vi "Lab Panel V5.40.vi"() -> ()   [LabVIEW 2017]
uses:
  sub vi/SelectLAB0X-N.ctl
  sub vi/SIG LAB0X-N.ctl
  sub vi/Set LAB0X-N.ctl
  <vilib>/Platform/TimedLoop/XDataNode/timing_clust.ctl
  <vilib>/Platform/TimedLoop/XDataNode/nitl_modes.ctl
  <vilib>/Platform/TimedLoop/XDataNode/wakeup.ctl
  Global display 1.vi
  Global display 4.vi
  Global display 3.vi
  Global display 2.vi
  Global 1.vi
  <vilib>/platform/TimedLoop/XDataNode/XDataNode.xnode
  <vilib>/Platform/TimedLoop/XDataNode/XDNodeRunTimeDep.lvlib
panel:
  in  "path to JPEG file":path=path "C:/Users/Mike/Documents/Crabtree/Crabtree/Hardware/crabtree"
  out "Simulate IND":bool
  out "Amb Tp":dbl format="%#.0f"
  out "Tp Up":dbl
  out "network error":bool
  out "TEMP":bool
  out "AI":bool
  in  "stop all":bool
  in  "ADMIN":bool
  in  "Tab Control 2":T1(tab)
  out "SIG LAB05-2":T2 {"PF" format="%.2f"; "AMPS" format="%.1f"}
  out "SIG LAB05-1":T2 {"PF" format="%.2f"; "AMPS" format="%.1f"}
  out "SIG LAB04-2":T2 {"PF" format="%.2f"; "AMPS" format="%.1f"}
  out "SIG LAB04-1":T2 {"PF" format="%.2f"; "AMPS" format="%.1f"}
  out "SIG LAB03-2":T2 {"PF" format="%.2f"; "AMPS" format="%.1f"}
  out "SIG LAB03-1":T2 {"PF" format="%.2f"; "AMPS" format="%.1f"}
  out "SIG LAB02-2":T2 {"PF" format="%.2f"; "AMPS" format="%.1f"}
  in  "RUN LAB01-1":bool
  in  "O/I  LAB05-1":bool
  in  "O/I  LAB05-2":bool
  in  "O/I  LAB04-1":bool
  in  "O/I  LAB04-2":bool
  in  "O/I  LAB02-1":bool
  in  "O/I  LAB02-2":bool
  in  "O/I  LAB01-2":bool
  in  "O/I  LAB01-1":bool
  in  "O/I  LAB03-1":bool
  in  "RUN LAB05-2":bool
  in  "RUN LAB05-1":bool
  in  "RUN LAB04-2":bool
  in  "RUN LAB04-1":bool
  in  "RUN LAB03-2":bool
  in  "RUN LAB03-1":bool
  in  "RUN LAB02-2":bool
  in  "RUN LAB02-1":bool
  in  "RUN LAB01-2":bool
  in  "SELECT LAB05-2":T3
  in  "SELECT LAB05-1":T3
  in  "SELECT LAB04-2":T3
  in  "SELECT LAB04-1":T3
  in  "SELECT LAB03-2":T3
  in  "SELECT LAB03-1":T3
  in  "SELECT LAB02-2":T3
  in  "SELECT LAB02-1":T3
  in  "SELECT LAB01-2":T3
  in  "SELECT LAB01-1":T3
  in  "O/I  LAB03-2":bool
  out "SIG LAB01-1":T2 {"PF" format="%.2f"; "AMPS" format="%.1f"}
  out "SIG LAB01-2":T2 {"PF" format="%.2f"; "AMPS" format="%.1f"}
  out "SIG LAB02-1":T2 {"PF" format="%.2f"; "AMPS" format="%.1f"}
  out "DISP LAB05-2":T4 {"MINS" format="%.2g"}
  out "DISP LAB05-1":T4 {"MINS" format="%.2g"}
  out "DISP LAB04-2":T4 {"MINS" format="%.2g"}
  out "DISP LAB04-1":T4 {"MINS" format="%.2g"}
  out "DISP LAB03-2":T4 {"MINS" format="%.2g"}
  out "DISP LAB03-1":T4 {"MINS" format="%.2g"}
  in  "SET LAB05-2":T5={"NAME"="", "DESCRIPTION"="", "CYCLES"=5.0, "T-RISE mins"=0.0, "T-RISE deg C"=0.0} {"CYCLES" min=5.0 step=1.0}
  in  "SET LAB05-1":T5={"NAME"="", "DESCRIPTION"="", "CYCLES"=5.0, "T-RISE mins"=0.0, "T-RISE deg C"=0.0} {"CYCLES" min=5.0 step=1.0}
  in  "SET LAB04-2":T5={"NAME"="", "DESCRIPTION"="", "CYCLES"=5.0, "T-RISE mins"=0.0, "T-RISE deg C"=0.0} {"CYCLES" min=5.0 step=1.0}
  in  "SET LAB04-1":T5={"NAME"="", "DESCRIPTION"="", "CYCLES"=5.0, "T-RISE mins"=0.0, "T-RISE deg C"=0.0} {"CYCLES" min=5.0 step=1.0}
  in  "SET LAB03-2":T5={"NAME"="", "DESCRIPTION"="", "CYCLES"=5.0, "T-RISE mins"=0.0, "T-RISE deg C"=0.0} {"CYCLES" min=5.0 step=1.0}
  in  "SET LAB03-1":T5={"NAME"="", "DESCRIPTION"="", "CYCLES"=5.0, "T-RISE mins"=0.0, "T-RISE deg C"=0.0} {"CYCLES" min=5.0 step=1.0}
  out "DISP LAB02-2":T4 {"MINS" format="%.2g"}
  out "DISP LAB02-1":T4 {"MINS" format="%.2g"}
  in  "SET LAB02-2":T5={"NAME"="", "DESCRIPTION"="", "CYCLES"=5.0, "T-RISE mins"=0.0, "T-RISE deg C"=0.0} {"CYCLES" min=5.0 step=1.0}
  in  "SET LAB02-1":T5={"NAME"="", "DESCRIPTION"="", "CYCLES"=5.0, "T-RISE mins"=0.0, "T-RISE deg C"=0.0} {"CYCLES" min=5.0 step=1.0}
  out "RESULT LAB05-2":bool
  out "RESULT LAB05-1":bool
  out "RESULT LAB04-2":bool
  out "RESULT LAB04-1":bool
  out "RESULT LAB03-2":bool
  out "RESULT LAB03-1":bool
  out "RESULT LAB02-2":bool
  out "RESULT LAB02-1":bool
  out "RESULT LAB01-2":bool
  out "RESULT LAB01-1":bool
  in  "SET LAB01-1":T6={"NAME"="", "DESCRIPTION"="", "CYCLES"=5.0, "T-RISE mins"=0.0, "T-RISE deg C"=0.0} {"CYCLES" min=5.0 step=1.0}
  in  "SET LAB01-2":T5={"NAME"="", "DESCRIPTION"="", "CYCLES"=5.0, "T-RISE mins"=0.0, "T-RISE deg C"=0.0} {"CYCLES" min=5.0 step=1.0}
  out "DISP LAB01-1":T4 {"MINS" format="%.2g"}
  out "DISP LAB01-2":T4 {"MINS" format="%.2f"}
  out "TEMP RISE LAB05-2":cluster{"TL":dbl, "TN":dbl}
  out "TEMP RISE LAB05-1":cluster{"TL":dbl, "TN":dbl}
  out "TEMP RISE LAB04-2":cluster{"TL":dbl, "TN":dbl}
  out "TEMP RISE LAB04-1":cluster{"TL":dbl, "TN":dbl}
  out "TEMP RISE LAB03-2":cluster{"TL":dbl, "TN":dbl}
  out "TEMP RISE LAB03-1":cluster{"TL":dbl, "TN":dbl}
  out "TEMP RISE LAB02-2":cluster{"TL":dbl, "TN":dbl}
  out "TEMP RISE LAB02-1":cluster{"TL":dbl, "TN":dbl}
  out "TEMP RISE LAB01-2":cluster{"TL":dbl, "TN":dbl}
  out "TEMP RISE LAB01-1":cluster{"TL":dbl, "TN":dbl}
  out "JIG LAB05-2":bool
  out "JIG LAB05-1":bool
  out "JIG LAB04-2":bool
  out "JIG LAB04-1":bool
  out "JIG LAB03-2":bool
  out "JIG LAB03-1":bool
  out "JIG LAB02-2":bool
  out "JIG LAB02-1":bool
  out "JIG LAB01-2":bool
  out "JIG LAB01-1":bool
  out "TEMP START LAB01-1":cluster{"TL":dbl, "TN":dbl}
  out "TEMP START LAB02-1":cluster{"TL":dbl, "TN":dbl}
  out "TEMP START LAB03-1":cluster{"TL":dbl, "TN":dbl}
  out "TEMP START LAB04-1":cluster{"TL":dbl, "TN":dbl}
  out "TEMP START LAB01-2":cluster{"TL":dbl, "TN":dbl}
  out "TEMP START LAB02-2":cluster{"TL":dbl, "TN":dbl}
  out "TEMP START LAB03-2":cluster{"TL":dbl, "TN":dbl}
  out "TEMP START LAB04-2":cluster{"TL":dbl, "TN":dbl}
  out "TEMP START LAB05-2":cluster{"TL":dbl, "TN":dbl}
  out "TEMP START LAB05-1":cluster{"TL":dbl, "TN":dbl}
  out "LOG LAB05-2":string
  out "LOG LAB04-2":string
  out "LOG LAB03-2":string
  out "LOG LAB02-2":string
  out "LOG LAB01-2":string
  out "LOG LAB05-1":string
  out "LOG LAB04-1":string
  out "LOG LAB03-1":string
  out "LOG LAB02-1":string
  out "LOG LAB01-1":string
  in  "Tab charts":T7(tab)
  out "LAB01 VOLTS":dynamicdata(graph)
  out "LAB01 AMPS":dynamicdata(graph)
  out "LAB01 deg C":dynamicdata(graph)
  out "LAB02 VOLTS":dynamicdata(graph)
  out "LAB02 AMPS":dynamicdata(graph)
  out "LAB02 deg C":dynamicdata(graph)
  out "LAB03 VOLTS":dynamicdata(graph)
  out "LAB03 AMPS":dynamicdata(graph)
  out "LAB03 deg C":dynamicdata(graph)
  out "LAB04 VOLTS":dynamicdata(graph)
  out "LAB04 AMPS":dynamicdata(graph)
  out "LAB04 deg C":dynamicdata(graph)
  out "LAB05 VOLTS":dynamicdata(graph)
  out "LAB05 AMPS":dynamicdata(graph)
  out "LAB05 deg C":dynamicdata(graph)
  out "Reset Error":bool
  out "Er USB#2":dbl
  out "Er USB#1":dbl
  out "Er USB#0":dbl
  out "Resets Done":dbl
  out "Error USB #2":bool
  out "Error USB #1":bool
  out "Error USB #0":bool
  in  "MAIL SETTINGS":T8
  out "MAIL REPORT":string
  in  "TO (string):":string
  in  "Send Mail Now":bool
  in  "Auto Mail Send":bool
  in  "Network Directory":path
  in  "JIG ON TIME (S)":dbl=1.0 min=1.0 max=10.0 step=0.5 format="%.1g"
  in  "JIG OFF TIME (S)":dbl=2.0 min=2.0 max=10.0 step=0.5 format="%.1g"
  in  "Reset Measuring":bool
  out "JIG RELAY CYCLES":T9
  out "ON L05-2":cluster{"amps":dbl, "volts":dbl, "pf":dbl}
  out "ON L05-1":cluster{"amps":dbl, "volts":dbl, "pf":dbl}
  out "FAIL LAB05-2":cluster{"LO":dbl, "HI":dbl}
  out "FAIL LAB05-1":cluster{"LO":dbl, "HI":dbl}
  out "FAIL LAB04-2":cluster{"LO":dbl, "HI":dbl}
  out "FAIL LAB04-1":cluster{"LO":dbl, "HI":dbl}
  out "FAIL LAB03-2":cluster{"LO":dbl, "HI":dbl}
  out "FAIL LAB03-1":cluster{"LO":dbl, "HI":dbl}
  out "FAIL LAB02-2":cluster{"LO":dbl, "HI":dbl}
  out "FAIL LAB02-1":cluster{"LO":dbl, "HI":dbl}
  out "FAIL LAB01-2":cluster{"LO":dbl, "HI":dbl}
  out "FAIL LAB01-1":cluster{"LO":dbl, "HI":dbl}
  out "ON L01-1":cluster{"amps":dbl, "volts":dbl, "pf":dbl}
  out "ON L01-2":cluster{"amps":dbl, "volts":dbl, "pf":dbl}
  out "ON L02-1":cluster{"amps":dbl, "volts":dbl, "pf":dbl}
  out "ON L02-2":cluster{"amps":dbl, "volts":dbl, "pf":dbl}
  out "ON L03-1":cluster{"amps":dbl, "volts":dbl, "pf":dbl}
  out "ON L03-2":cluster{"amps":dbl, "volts":dbl, "pf":dbl}
  out "ON L04-1":cluster{"amps":dbl, "volts":dbl, "pf":dbl}
  out "ON L04-2":cluster{"amps":dbl, "volts":dbl, "pf":dbl}
  in  "Open Com Port":bool
  out "LA05-2 (TN)":bool
  out "LA05-2 (TL)":bool
  out "LA05-1 (TN)":bool
  out "LA05-1 (TL)":bool
  out "LA04-2 (TN)":bool
  out "LA04-2 (TL)":bool
  out "LA04-1 (TN)":bool
  out "LA04-1 (TL)":bool
  out "LA03-2 (TN)":bool
  out "LA03-2 (TL)":bool
  out "LA03-1 (TN)":bool
  out "LA03-1 (TL)":bool
  out "LA02-2 (TN)":bool
  out "LA02-2 (TL)":bool
  out "LA02-1 (TN)":bool
  out "LA02-1 (TL)":bool
  out "LA01-2 (TN)":bool
  out "LA01-2 (TL)":bool
  out "LA01-1 (TN)":bool
  out "LA01-1 (TL)":bool
  out "TEMP LA05":T10
  out "TEMP LA04":T10
  out "TEMP LA03":T10
  out "TEMP LA02":T10
  out "TEMP LA01":T10
  out "Ref deg C":dbl format="%#.0f"
  out "Temp read loop":dbl
  out "Com Port Status":bool
  out "Com setup loops":i32
  out "VISA Com out":refnum<visa-resource-name>
  in  "Select COM port":refnum<visa-resource-name>="COM6"
  in  "Read Temp":bool
  out "Error Temp":bool
  out "AI Task":bool
  out "AI Task2":dbl
  out "AI Task1":dbl
  out "AI Task0":dbl
  out "Total USB resets":dbl
  in  "Auto Reset":bool
  in  "Mail Test File To:":string
  in  "Mail Test Fail":bool
  out "graph flag":bool
  in  "Temp Test Cal":dbl
  in  "Amps Fail level":dbl
  in  "Fail Loops":dbl
  out "Save JC":bool
  in  "Simulate":bool
  in  "Temp Value":dbl
  in  "Temp Delay Lps":dbl
  in  "SAMPLES":dbl
  in  "RATE (Hz)":dbl
  in  "JIG TEST":T11
  in  "C drive data root dir":path
  out "run lab05-2":bool
  out "run lab05-1":bool
  out "run lab04-2":bool
  out "run lab04-1":bool
  out "run lab03-2":bool
  out "run lab03-1":bool
  out "run lab02-2":bool
  out "run lab02-1":bool
  out "run lab01-2":bool
  out "run lab01-1":bool
  in  "Tab Control":T12(tab)
  out "LAB01-2 (GRAPH)":dynamicdata(graph)
  out "LAB01-1 (GRAPH)":dynamicdata(graph)
  out "LAB02-2 (GRAPH)":dynamicdata(graph)
  out "LAB02-1 (GRAPH)":dynamicdata(graph)
  out "LAB03-2 (GRAPH)":dynamicdata(graph)
  out "LAB03-1 (GRAPH)":dynamicdata(graph)
  out "LAB04-2 (GRAPH)":dynamicdata(graph)
  out "LAB04-1 (GRAPH)":dynamicdata(graph)
  out "LAB05-2 (GRAPH)":dynamicdata(graph)
  out "LAB05-1 (GRAPH)":dynamicdata(graph)
  out "Any Test Running":bool
  out "Read Time":dbl
  out "LAB05 TEMP":T13
  out "LAB04 TEMP":T13
  out "LAB02 TEMP":T13
  out "LAB01 TEMP":T13
  out "LAB03 TEMP":T13
  out "LAB05-TP":bool
  out "LAB04-TP":bool
  out "LAB03-TP":bool
  out "LAB02-TP":bool
  out "LAB01-TP":bool
  out "Analog error":bool
  out "USB OUT 0":bool[](array[boolean])
  out "USB OUT 1":bool[](array[boolean])
  out "USB OUT 2":bool[](array[boolean])
  in  "Ambient Volts":dbl format="%.2f"
  in  "PF":dbl min=0.0 max=1.0 step=0.1 format="%#.1f"
  in  "VOLTS":dbl
  in  "OFF amps":dbl min=0.0 max=100.0 step=0.1 format="%#.1f"
  in  "ON amps":dbl
  in  "LAB deg C":T14
  out "AI data 0":waveform(dbl)[](array[waveform])
  out "AI data 1":waveform(dbl)[](array[waveform])
  out "AI data 2":waveform(dbl)[](array[waveform])
  out "AI Error":errorcluster[](array[cluster])
  out "AI loop time":dbl format="%.6g"
  out "loops":dbl
  out "on loops":dbl format="%#.0f"
  out "off loops":dbl format="%#.0f"
  out "jig cycle":dbl
  out "TDMS LAB01-1":refnum<k34>
  out "data file error":errorcluster
  out "TDMS LAB02-1":refnum<k34>
  out "TDMS LAB01-2":refnum<k34>
  out "TDMS LAB02-2":refnum<k34>
  out "TDMS LAB03-1":refnum<k34>
  out "TDMS LAB03-2":refnum<k34>
  out "TDMS LAB04-1":refnum<k34>
  out "TDMS LAB04-2":refnum<k34>
  out "TDMS LAB05-1":refnum<k34>
  out "TDMS LAB05-2":refnum<k34>
  out "mail control":string
  out "File Time Stamp":timestamp
  in  "stop":bool
  out "deg C (volts)":dbl
  out "TEMP REF cal":dbl
  out "CAL LAB01":T15 {"2 (TN) cal" min=0.0 step=0.01 format="%.2f"; "2 (TL) cal" min=0.0 step=0.01 format="%.2f"; "2 (PF) cal" min=0.0 step=0.01 format="%.2f"; "2 (V) cal" min=0.0 step=0.01 format="%.2f"; "2 (A) cal" min=0.0 step=0.01 format="%.2f"; "1 (TN) cal" min=0.0 step=0.01 format="%.2f"; "1 (TL) cal" min=0.0 step=0.01 format="%.2f"; "1 (PF) cal" min=0.0 step=0.01 format="%.2f"; "1 (V) cal" min=0.0 step=0.01 format="%.2f"; "1  (A) cal" min=0.0 step=0.01 format="%.2f"}
  out "CAL LAB03":T15 {"2 (TN) cal" min=0.0 step=0.01 format="%.2f"; "2 (TL) cal" min=0.0 step=0.01 format="%.2f"; "2 (PF) cal" min=0.0 step=0.01 format="%.2f"; "2 (V) cal" min=0.0 step=0.01 format="%.2f"; "2 (A) cal" min=0.0 step=0.01 format="%.2f"; "1 (TN) cal" min=0.0 step=0.01 format="%.2f"; "1 (TL) cal" min=0.0 step=0.01 format="%.2f"; "1 (PF) cal" min=0.0 step=0.01 format="%.2f"; "1 (V) cal" min=0.0 step=0.01 format="%.2f"; "1  (A) cal" min=0.0 step=0.01 format="%.2f"}
  out "CAL LAB02":T16 {"2 (TN) cal" min=0.0 step=0.01 format="%.2f"; "2 (TL) cal" min=0.0 step=0.01 format="%.2f"; "2 (PF) cal" min=0.0 step=0.01 format="%.2f"; "2 (V) cal" min=0.0 step=0.01 format="%.2f"; "2 (A) cal" min=0.0 step=0.01 format="%.2f"; "1 (TN) cal" min=0.0 step=0.01 format="%.2f"; "1 (TL) cal" min=0.0 step=0.01 format="%.2f"; "1 (PF) cal" min=0.0 step=0.01 format="%.2f"; "1 (V) cal" min=0.0 step=0.01 format="%.2f"; "1 (A) cal" min=0.0 step=0.01 format="%.2f"}
  out "CAL LAB05":T15 {"2 (TN) cal" min=0.0 step=0.01 format="%.2f"; "2 (TL) cal" min=0.0 step=0.01 format="%.2f"; "2 (PF) cal" min=0.0 step=0.01 format="%.2f"; "2 (V) cal" min=0.0 step=0.01 format="%.2f"; "2 (A) cal" min=0.0 step=0.01 format="%.2f"; "1 (TN) cal" min=0.0 step=0.01 format="%.2f"; "1 (TL) cal" min=0.0 step=0.01 format="%.2f"; "1 (PF) cal" min=0.0 step=0.01 format="%.2f"; "1 (V) cal" min=0.0 step=0.01 format="%.2f"; "1  (A) cal" min=0.0 step=0.01 format="%.2f"}
  out "CAL LAB04":T15 {"2 (TN) cal" min=0.0 step=0.01 format="%.2f"; "2 (TL) cal" min=0.0 step=0.01 format="%.2f"; "2 (PF) cal" min=0.0 step=0.01 format="%.2f"; "2 (V) cal" min=0.0 step=0.01 format="%.2f"; "2 (A) cal" min=0.0 step=0.01 format="%.2f"; "1 (TN) cal" min=0.0 step=0.01 format="%.2f"; "1 (TL) cal" min=0.0 step=0.01 format="%.2f"; "1 (PF) cal" min=0.0 step=0.01 format="%.2f"; "1 (V) cal" min=0.0 step=0.01 format="%.2f"; "1  (A) cal" min=0.0 step=0.01 format="%.2f"}
  out "cal file error out":errorcluster
  in  "SET (cal)":bool
  out "AI Data 0":waveform(dbl)[](graph)
  out "AI Data 1":waveform(dbl)[](graph)
  out "AI Data 2":waveform(dbl)[](graph)
  # "LAB01"
  # "LAB02"
  # "LAB03"
  # "LAB04"
  # "LAB05"
  # "LAB01"
  # "LAB02"
  # "LAB03"
  # "LAB04"
  # "LAB05"
  # "PANEL ID / DATE / TIME / NAME / DESCRIPTION / CYCLES / TEST TIME / STATUS"
  # "PANEL ID / DATE / TIME / NAME / DESCRIPTION / CYCLES / TEST TIME / STATUS"
  # "(Enter recipients address seperated by comma)"
  # "JIG SET"
  # "Temperature circuits \ndetected at start up."
  # "PANEL CONTROL TO BE ON"
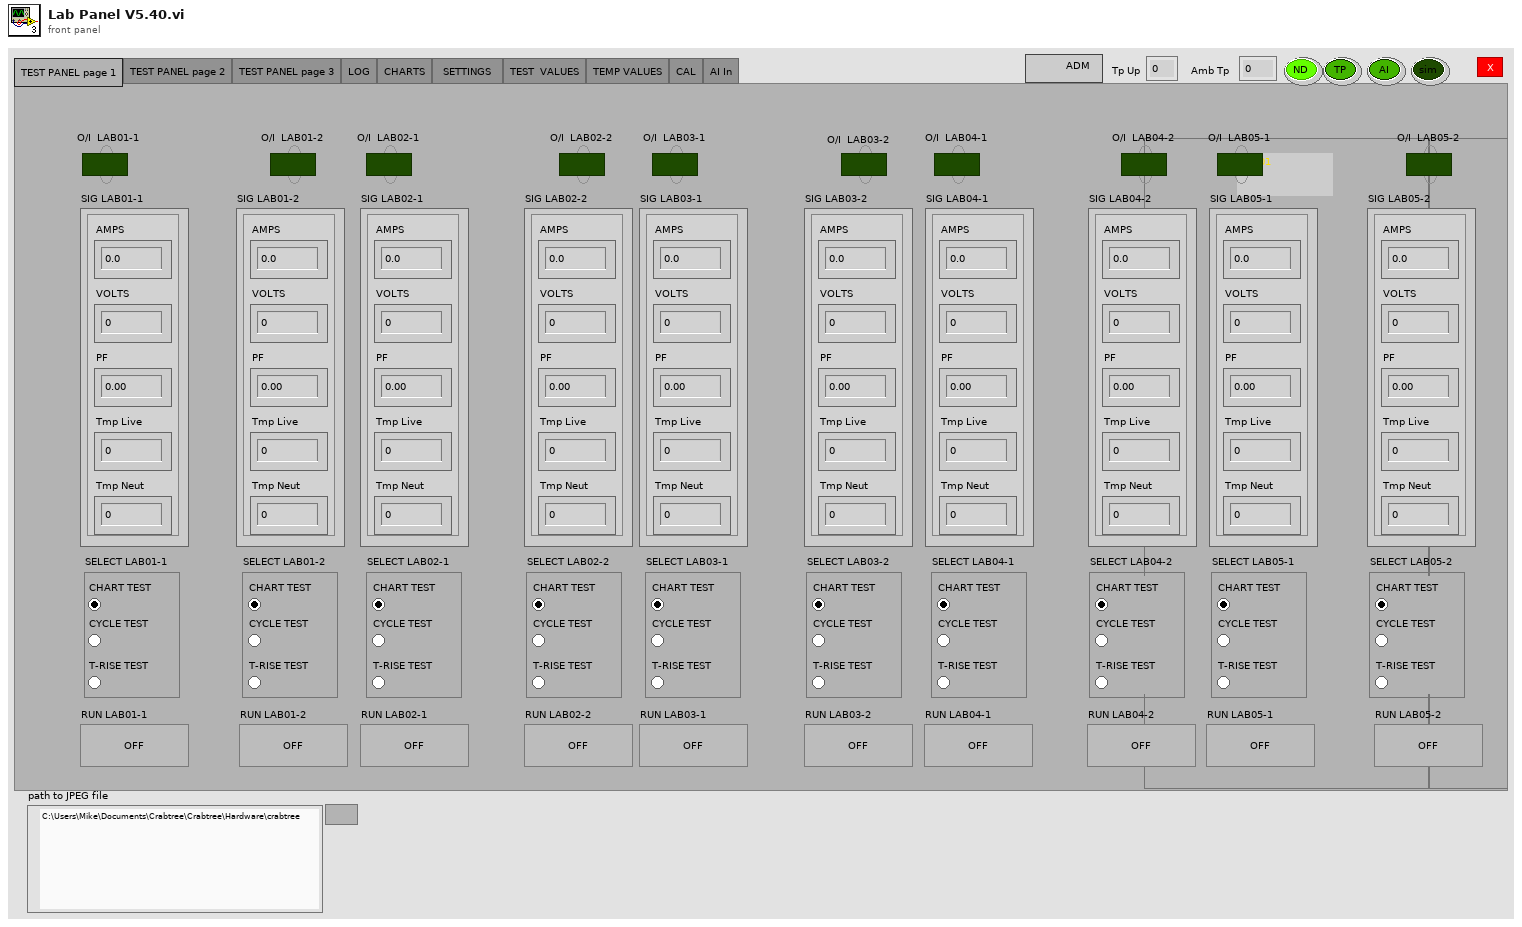
[diagram p1: front panel]
types:
  T1 = enum32{"TEST PANEL page 1", "TEST PANEL page 2", "TEST PANEL page 3", "LOG", "CHARTS", "SETTINGS   ", "TEST  VALUES", "TEMP VALUES", "ADM", "CAL", "AI In"}
  T2 = typedef "SIG LAB0X-N.ctl" = cluster{"AMPS":dbl, "VOLTS":dbl, "PF":dbl, "Tmp Live":dbl, "Tmp Neut":dbl}
  T3 = typedef "SelectLAB0X-N.ctl" = enum32{"CHART TEST", "CYCLE TEST", "T-RISE TEST"}
  T4 = cluster{"CYCLE":dbl, "MINS":dbl, "STATUS":string}
  T5 = cluster{"NAME":string, "DESCRIPTION":string, "CYCLES":dbl, "T-RISE mins":dbl, "T-RISE deg C":dbl}
  T6 = typedef "Set LAB0X-N.ctl" = cluster{"NAME":string, "DESCRIPTION":string, "CYCLES":dbl, "T-RISE mins":dbl, "T-RISE deg C":dbl}
  T7 = enum32{"LAB01", "LAB02", "LAB03", "LAB04", "LAB05"}
  T8 = cluster{"OUT SERVER ADDRESS":string, "FROM ACCOUNT":string, "USER NAME":string, "PASSWORD":string, "TEST MAIL":bool, "TEST MAIL STATUS":string, "mail error":errorcluster}
  T9 = cluster{"LAB01-1":dbl, "LAB01-2":dbl, "LAB02-1":dbl, "LAB02-2":dbl, "LAB03-1":dbl, "LAB03-2":dbl, "LAB04-1":dbl, "LAB04-2":dbl, "LAB05-1":dbl, "LAB05-2":dbl}
  T10 = cluster{"TL-1":dbl, "TN-1":dbl, "TL-2":dbl, "TN-2":dbl, "TL -1COUNT":dbl, "TN-1 COUNT":dbl, "TL-2 COUNT":dbl, "TN-2 COUNT":dbl}
  T11 = cluster{" LAB01-1":bool, " LAB01-2":bool, "LAB02-1":bool, " LAB02-2":bool, "LAB03-1":bool, "LAB03-2":bool, "LAB04-1":bool, "LAB04-2":bool, "LAB05-1":bool, "LAB05-2":bool}
  T12 = enum32{"LAB01", "LAB02", "LAB03", "LAB04", "LAB05", "TEMPERATURE", "GENERAL INFO", "Simulate", "AI Data Out"}
  T13 = cluster{"T1 Live":dbl, "T1 Neut":dbl, "T2 Live":dbl, "T2 Neut":dbl, "ID":dbl, "ER":dbl}
  T14 = cluster{"1 TL":dbl, "1 TN":dbl, "2 TL":dbl, "2 TN":dbl, "ID":dbl, "ER":dbl}
  T15 = cluster{"1  (A) cal":dbl, "1 (V) cal":dbl, "1 (PF) cal":dbl, "1 (TL) cal":dbl, "1 (TN) cal":dbl, "2 (A) cal":dbl, "2 (V) cal":dbl, "2 (PF) cal":dbl, "2 (TL) cal":dbl, "2 (TN) cal":dbl}
  T16 = cluster{"1 (A) cal":dbl, "1 (V) cal":dbl, "1 (PF) cal":dbl, "1 (TL) cal":dbl, "1 (TN) cal":dbl, "2 (A) cal":dbl, "2 (V) cal":dbl, "2 (PF) cal":dbl, "2 (TL) cal":dbl, "2 (TN) cal":dbl}
  T17 = enum8{"Enabled", "Disabled", "Disabled and Grayed Out"}
  T18 = enum16{"open", "replace", "create", "open or create", "replace or create", "replace or create with confirmation"}
  T19 = typedef "XDNodeRunTimeDep.lvlib/timing_clust.ctl" = cluster{"Expected End [f-1]":u64, "Actual End [f-1]":u64, "Finished Late? [f-1]":bool, "Expected End [i-1]":u64, "Actual End [i-1]":u64, "Finished Late? [i-1]":bool, "Expected Start [i]":u64, "Actual Start [i]":u64, "Expected Start [f]":u64, "Actual Start [f]":u64, "Source Name":string, "Structure Name":string, "Period":i64, "Deadline":i64, "Offset":i64, "Start":i64, "Priority":i32, "Timeout":i32, "Mode":T20, "Wakeup Reason":T21, "Error":errorcluster, "Source Type":string, "Secondary Source Type":string, "Global End Time":u64, "Global Start Time":u64, "Frame Duration":u64, "Iteration Duration":u64, "Assigned CPU":i32, "I/O Scan Engine Mode":u32}
  T20 = typedef "XDNodeRunTimeDep.lvlib/nitl_modes.ctl" = enum32{"No Change", "Process missed periods, maintain original phase", "Discard missed periods, maintain original phase", "Process missed periods, ignore original phase", "Discard missed periods, ignore original phase"}
  T21 = typedef "XDNodeRunTimeDep.lvlib/wakeup.ctl" = enum32{"Normal", "Aborted", "Asynchronous wakeup", "Timing source error", "Timed loop error", "Timeout"}
  T22 = enum16{"open", "open or create", "create or replace", "create", "open (read-only)"}
  T23 = cluster{"status":string, "mail server":string, "mail from":string, "mail to":string, "mail file":bool}
  T24 = cluster{"SET LAB01-1":T6, "SET LAB01-2":cluster{"NAME":string, "DESCRIPTION":string, "CYCLES":dbl, "T-RISE mins":dbl, "T-RISE deg C":dbl}, "SET LAB02-1":cluster{"NAME":string, "DESCRIPTION":string, "CYCLES":dbl, "T-RISE mins":dbl, "T-RISE deg C":dbl}, "SET LAB02-2":cluster{"NAME":string, "DESCRIPTION":string, "CYCLES":dbl, "T-RISE mins":dbl, "T-RISE deg C":dbl}, "SET LAB03-1":cluster{"NAME":string, "DESCRIPTION":string, "CYCLES":dbl, "T-RISE mins":dbl, "T-RISE deg C":dbl}, "SET LAB03-2":cluster{"NAME":string, "DESCRIPTION":string, "CYCLES":dbl, "T-RISE mins":dbl, "T-RISE deg C":dbl}, "SET LAB04-1":cluster{"NAME":string, "DESCRIPTION":string, "CYCLES":dbl, "T-RISE mins":dbl, "T-RISE deg C":dbl}, "SET LAB04-2":cluster{"NAME":string, "DESCRIPTION":string, "CYCLES":dbl, "T-RISE mins":dbl, "T-RISE deg C":dbl}, "SET LAB05-1":cluster{"NAME":string, "DESCRIPTION":string, "CYCLES":dbl, "T-RISE mins":dbl, "T-RISE deg C":dbl}, "SET LAB05-2":cluster{"NAME":string, "DESCRIPTION":string, "CYCLES":dbl, "T-RISE mins":dbl, "T-RISE deg C":dbl}, "Network Directory":path, "C drive data root dir":path, "RATE (Hz)":dbl, "SAMPLES":dbl, "Select COM port":refnum<visa-resource-name>, "Temp Delay Lps":dbl, "Temp Value":dbl, "Fail Loops":dbl, "Temp Test Cal":dbl, "Amps Fail level":dbl, "Mail Test File To:":string, "Mail Test Fail":bool}
  T25 = cluster{"MAIL SETTINGS":cluster{"OUT SERVER ADDRESS":string, "FROM ACCOUNT":string, "USER NAME":string, "PASSWORD":string, "TEST MAIL":bool, "TEST MAIL STATUS":string, "mail error":errorcluster}, "Auto Mail Send":bool, string}
  T26 = cluster{"id1":bool, "id2":bool, "id3":bool, "id4":bool, "id5":bool}
  T27 = cluster{"T1":dbl, "T2":dbl, "T3":dbl, "T4":dbl, "ID":dbl, "ER":dbl}
  T28 = typedef "imagedata.ctl" = cluster{"image type":i32, "image depth":i32, "image":u8[], "mask":u8[], "colors":u32[], "Rectangle":cluster{"left":i16, "top":i16, "right":i16, "bottom":i16}}
  T29 = cluster{"STATUS":string, "OUT SERVER ADDRESS":string, "FROM ACCOUNT":string, "Mail Test File To:":string, "Mail Test Fail":bool}
  T30 = cluster{"LAB01-1 (A)":dbl, "LAB01-1 (V)":dbl, "LAB01-1 (PF)":dbl, "LAB01-2 (A)":dbl, "LAB01-2 (V)":dbl, "LAB01-2 (PF)":dbl}
  T31 = cluster{"LAB02-1 (A)":dbl, "LAB02-1 (V)":dbl, "LAB02-1 (PF)":dbl, "LAB02-2 (A)":dbl, "LAB02-2 (V)":dbl, "LAB02-2 (PF)":dbl}
  T32 = cluster{"LAB03-1 (A)":dbl, "LAB03-1 (V)":dbl, "LAB03-1 (PF)":dbl, "LAB03-2 (A)":dbl, "LAB03-2 (V)":dbl, "LAB03-2 (PF)":dbl}
  T33 = cluster{"LAB04-1 (A)":dbl, "LAB04-1 (V)":dbl, "LAB04-1 (PF)":dbl, "LAB04-2 (A)":dbl, "LAB04-2 (V)":dbl, "LAB04-2 (PF)":dbl}
  T34 = cluster{"LAB05-1 (A)":dbl, "LAB05-1 (V)":dbl, "LAB05-1 (PF)":dbl, "LAB05-2 (A)":dbl, "LAB05-2 (V)":dbl, "LAB05-2 (PF)":dbl}
  T35 = cluster{"OFF amps":dbl, "VOLTS":dbl, "PF":dbl, "OFF amps":dbl, "VOLTS":dbl, "PF":dbl}
  T36 = cluster{"FAIL LAB01-1":cluster{"LO":dbl, "HI":dbl}, "SIG LAB01-1":T2, "TEMP START LAB01-1":cluster{"TL":dbl, "TN":dbl}, "DISP LAB01-1":cluster{"CYCLE":dbl, "MINS":dbl, "STATUS":string}, "SET LAB01-1":T6, "TDMS LAB01-1":refnum<k34>}
  T37 = cluster{"FAIL LAB01-2":cluster{"LO":dbl, "HI":dbl}, "SIG LAB01-2":T2, "TEMP START LAB01-2":cluster{"TL":dbl, "TN":dbl}, "DISP LAB01-2":cluster{"CYCLE":dbl, "MINS":dbl, "STATUS":string}, "SET LAB01-2":cluster{"NAME":string, "DESCRIPTION":string, "CYCLES":dbl, "T-RISE mins":dbl, "T-RISE deg C":dbl}, "TDMS LAB01-2":refnum<k34>}
  T38 = cluster{"FAIL LAB02-1":cluster{"LO":dbl, "HI":dbl}, "SIG LAB02-1":T2, "TEMP START LAB02-1":cluster{"TL":dbl, "TN":dbl}, "DISP LAB02-1":cluster{"CYCLE":dbl, "MINS":dbl, "STATUS":string}, "SET LAB02-1":cluster{"NAME":string, "DESCRIPTION":string, "CYCLES":dbl, "T-RISE mins":dbl, "T-RISE deg C":dbl}, "TDMS LAB02-1":refnum<k34>}
  T39 = cluster{"FAIL LAB02-2":cluster{"LO":dbl, "HI":dbl}, "SIG LAB02-2":T2, "TEMP START LAB02-2":cluster{"TL":dbl, "TN":dbl}, "DISP LAB02-2":cluster{"CYCLE":dbl, "MINS":dbl, "STATUS":string}, "SET LAB02-2":cluster{"NAME":string, "DESCRIPTION":string, "CYCLES":dbl, "T-RISE mins":dbl, "T-RISE deg C":dbl}, "TDMS LAB02-2":refnum<k34>}
  T40 = cluster{"FAIL LAB03-1":cluster{"LO":dbl, "HI":dbl}, "SIG LAB03-1":T2, "TEMP START LAB03-1":cluster{"TL":dbl, "TN":dbl}, "DISP LAB03-1":cluster{"CYCLE":dbl, "MINS":dbl, "STATUS":string}, "SET LAB03-1":cluster{"NAME":string, "DESCRIPTION":string, "CYCLES":dbl, "T-RISE mins":dbl, "T-RISE deg C":dbl}, "TDMS LAB03-1":refnum<k34>}
  T41 = cluster{"FAIL LAB03-2":cluster{"LO":dbl, "HI":dbl}, "SIG LAB03-2":T2, "TEMP START LAB03-2":cluster{"TL":dbl, "TN":dbl}, "DISP LAB03-2":cluster{"CYCLE":dbl, "MINS":dbl, "STATUS":string}, "SET LAB03-2":cluster{"NAME":string, "DESCRIPTION":string, "CYCLES":dbl, "T-RISE mins":dbl, "T-RISE deg C":dbl}, "TDMS LAB03-2":refnum<k34>}
  T42 = cluster{"FAIL LAB04-1":cluster{"LO":dbl, "HI":dbl}, "SIG LAB04-1":T2, "TEMP START LAB04-1":cluster{"TL":dbl, "TN":dbl}, "DISP LAB04-1":cluster{"CYCLE":dbl, "MINS":dbl, "STATUS":string}, "SET LAB04-1":cluster{"NAME":string, "DESCRIPTION":string, "CYCLES":dbl, "T-RISE mins":dbl, "T-RISE deg C":dbl}, "TDMS LAB04-1":refnum<k34>}
  T43 = cluster{"FAIL LAB04-2":cluster{"LO":dbl, "HI":dbl}, "SIG LAB04-2":T2, "TEMP START LAB04-2":cluster{"TL":dbl, "TN":dbl}, "DISP LAB04-2":cluster{"CYCLE":dbl, "MINS":dbl, "STATUS":string}, "SET LAB04-2":cluster{"NAME":string, "DESCRIPTION":string, "CYCLES":dbl, "T-RISE mins":dbl, "T-RISE deg C":dbl}, "TDMS LAB04-2":refnum<k34>}
  T44 = cluster{"FAIL LAB05-1":cluster{"LO":dbl, "HI":dbl}, "SIG LAB05-1":T2, "TEMP START LAB05-1":cluster{"TL":dbl, "TN":dbl}, "DISP LAB05-1":cluster{"CYCLE":dbl, "MINS":dbl, "STATUS":string}, "SET LAB05-1":cluster{"NAME":string, "DESCRIPTION":string, "CYCLES":dbl, "T-RISE mins":dbl, "T-RISE deg C":dbl}, "TDMS LAB05-1":refnum<k34>}
  T45 = cluster{"FAIL LAB05-2":cluster{"LO":dbl, "HI":dbl}, "SIG LAB05-2":T2, "TEMP START LAB05-2":cluster{"TL":dbl, "TN":dbl}, "DISP LAB05-2":cluster{"CYCLE":dbl, "MINS":dbl, "STATUS":string}, "SET LAB05-2":cluster{"NAME":string, "DESCRIPTION":string, "CYCLES":dbl, "T-RISE mins":dbl, "T-RISE deg C":dbl}, "TDMS LAB05-2":refnum<k34>}
  T46 = cluster{"MAIL SETTINGS":cluster{"OUT SERVER ADDRESS":string, "FROM ACCOUNT":string, "USER NAME":string, "PASSWORD":string, "TEST MAIL":bool, "TEST MAIL STATUS":string, "mail error":errorcluster}, "Auto Mail Send":bool, "TO (string):":string}
  T47 = cluster{"TP1-L":dbl, "TP1-N":dbl, "TP2-L":dbl, "TP2-N":dbl, "TP1-L COUNT":dbl, "TP1-N COUNT":dbl, "TP2-L COUNT":dbl, "TP2-N COUNT":dbl}
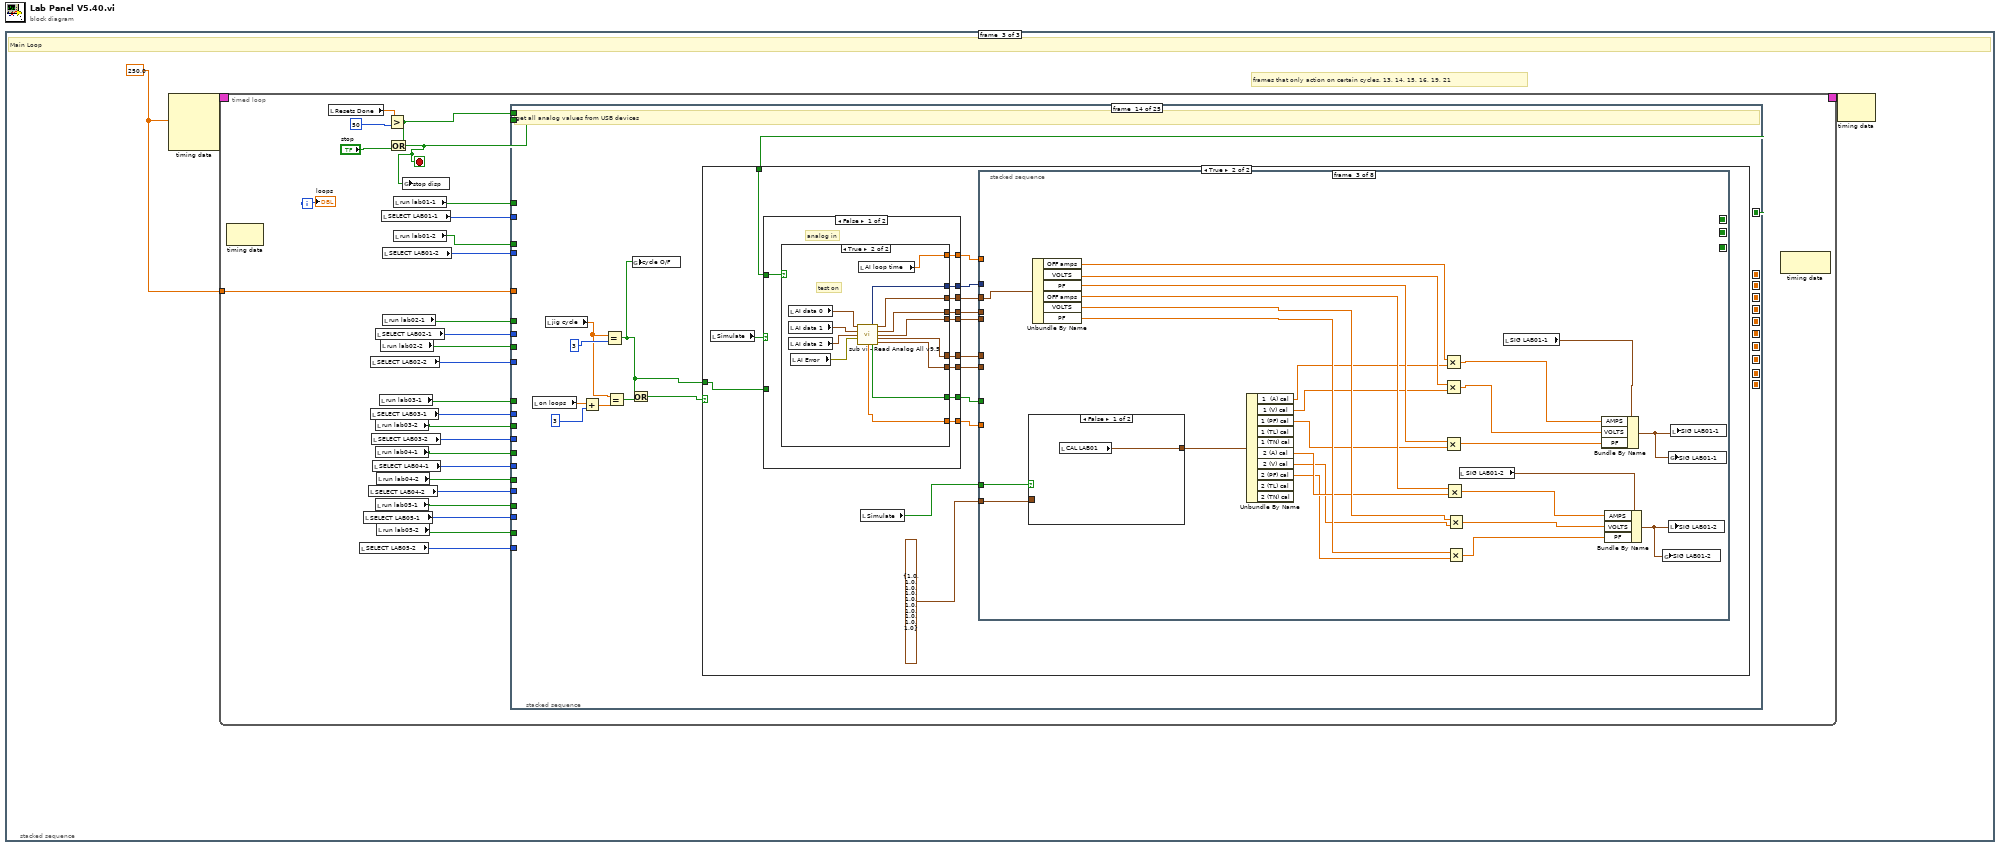
[diagram p0: block diagram]
diagram:
  n1 = stacked-sequence {
    frame #0 {
      n2 = local write "Save JC"(FALSE) -> ()
      "jig cycle" <- 0
    }
    frame #1 {
      # "do 1st time set up"
      n3 = stacked-sequence {
        frame #0 {
          # "check for simulate mode"
          n4 = call "subvi-simulate v1.vi"() -> ("Sim"=w3:bool)  [unwired: 11 in]
          n5 = case shown="True" w3 {
            frame False {
            }
            frame True {
              n6 = local write "Simulate"(TRUE) -> ()
            }
          }
        }
        frame #1 {
          # "RESET USB AND TEMPERATURE CIRCUITS"
          n7 = local read "Simulate"() -> (w5:bool)
          n8 = case shown="False" w5 {
            frame False {
              n9 = call "Reset USB&temp v 1.vi"() -> ()  [unwired: 11 in, 1 out]
            }
            frame True {
            }
          }
        }
        frame #2 {
          # "Disable front panel while 1st time set up is being done"
          n10 = disable-structure shown="Enabled" {
            frame Enabled {
              n11 = property on="Tab Control 2" class="TabCtl (strict)"() -> ("Pages"=w12:refnum<vi>[])  [unwired: 2 in, 2 out]
              n12 = Index Array(array=w12, index=8) -> (element=w10:refnum<vi>)
              n13 = property class="Page"(reference=w10, "PageVis"=FALSE) -> ()  [unwired: 1 in, 2 out]
            }
            frame Disabled {
            }
          }
          n14 = property on="Tab Control 2" class="TabCtl (strict)"("Value"=0) -> ()  [unwired: 2 in, 2 out]
          n15 = local write "ADMIN"(FALSE) -> ()
          n16 = property on="Tab Control 2" class="TabCtl (strict)"("DisabledEnum"=T17."Disabled and Grayed Out" ("Disabled")) -> ()  [unwired: 2 in, 2 out]
        }
        frame #3 {
          # "Get calibration values"
          n17 = call "sub vi - get calibration values v1.vi"() -> ("TEMP REF CAL"=w13:dbl, "LAB01 (CAL)"=→"CAL LAB01":T15, "LAB02 (CAL)"=→"CAL LAB02":T16, "LAB03 (CAL)"=→"CAL LAB03":T15, "LAB04 (CAL)"=→"CAL LAB04":T15, "calibration file error out"=→"cal file error out":errorcluster, "LAB05 (CAL)"=→"CAL LAB05":T15)  [unwired: 9 in]
          n18 = local write "TEMP REF cal"(w13) -> ()
        }
        frame #4 {
          # "get last saved test settings from file"
          n19 = local read "Network Directory"() -> (w42:path)
          n20 = local read "C drive data root dir"() -> (w40:path)
          n21 = local read "SET LAB05-2"() -> (w72:T5)
          n22 = local read "SAMPLES"() -> (w38:dbl)
          n23 = local read "SET LAB05-1"() -> (w73:T5)
          n24 = local read "RATE (Hz)"() -> (w39:dbl)
          n25 = local read "SET LAB04-2"() -> (w74:T5)
          n26 = local read "SET LAB03-2"() -> (w71:T5)
          n27 = local read "SET LAB04-1"() -> (w75:T5)
          n28 = local read "SET LAB03-1"() -> (w70:T5)
          n29 = local read "SET LAB02-2"() -> (w69:T5)
          n30 = local read "SET LAB02-1"() -> (w68:T5)
          n31 = local read "SET LAB01-2"() -> (w67:T5)
          n32 = local read "SET LAB01-1"() -> (w66:T6)
          n33 = local read "Select COM port"() -> (w35:refnum<visa-resource-name>)
          n34 = local read "Temp Delay Lps"() -> (w34:dbl)
          n35 = local read "Mail Test File To:"() -> (w24:string)
          n36 = local read "Temp Value"() -> (w33:dbl)
          n37 = local read "Temp Test Cal"() -> (w28:dbl)
          n38 = local read "Amps Fail level"() -> (w27:dbl)
          n39 = local read "Fail Loops"() -> (w30:dbl)
          n40 = local read "Mail Test Fail"() -> (w22:bool)
          n41 = Bundle("SET LAB01-1"=w66, "SET LAB01-2"=w67, "SET LAB02-1"=w68, "SET LAB02-2"=w69, "SET LAB03-1"=w70, "SET LAB03-2"=w71, "SET LAB04-1"=w75, "SET LAB04-2"=w74, "SET LAB05-1"=w73, "SET LAB05-2"=w72, "Network Directory"=w42, "C drive data root dir"=w40, "RATE (Hz)"=w39, "SAMPLES"=w38, "Select COM port"=w35, "Temp Delay Lps"=w34, "Temp Value"=w33, "Fail Loops"=w30, "Temp Test Cal"=w28, "Amps Fail level"=w27, "Mail Test File To:"=w24, "Mail Test Fail"=w22) -> (w59:T24)  [unwired: 1 in]
          n42 = String To Path(string="c:\\crabtree\\Set Up\\") -> (path=w63:path)
          n43 = Build Path(base path=w63, name or relative path="settings.bin") -> (appended path=w61:path)
          n44 = Create Folder(path (use dialog)=w63) -> (error out=w65:errorcluster)  [unwired: 2 in, 2 out]
          n45 = call <vilib>:"Clear Errors.vi"("error in (no error)"=w65) -> ()  [unwired: 5 in, 2 out]
          n46 = Open/Create/Replace File(file path (use dialog)=w61) -> (refnum out=w58:refnum<file>, error out=w60:errorcluster)  [unwired: 5 in, 1 out]
          n47 = Read from Binary File(5:w59, 8:w60, 11:w58) -> (0:w55:errorcluster, 2:w57:T24, 3:w56:refnum<file>)  [unwired: 3 in, 1 out]
          n48 = Unbundle(w57) -> ("SET LAB01-1"=w53:T6, "SET LAB01-2"=w52:T5, "SET LAB02-1"=w51:T5, "SET LAB02-2"=w50:T5, "SET LAB03-1"=w49:T5, "SET LAB03-2"=w48:T5, "SET LAB04-1"=w47:T5, "SET LAB04-2"=w46:T5, "SET LAB05-1"=w45:T5, "SET LAB05-2"=w44:T5, "Network Directory"=w43:path, "C drive data root dir"=w41:path, "RATE (Hz)"=w36:dbl, "SAMPLES"=w37:dbl, "Select COM port"=w20:refnum<visa-resource-name>, "Temp Delay Lps"=w32:dbl, "Temp Value"=w31:dbl, "Fail Loops"=w29:dbl, "Temp Test Cal"=w26:dbl, "Amps Fail level"=w25:dbl, "Mail Test File To:"=w23:string, "Mail Test Fail"=w21:bool)
          n49 = Close File(refnum=w56, error in=w55) -> (error out=w54:errorcluster)  [unwired: 1 out]
          n50 = local write "data file error"(w54) -> ()
          n51 = local write "Temp Test Cal"(w26) -> ()
          n52 = local write "Amps Fail level"(w25) -> ()
          n53 = local write "Mail Test File To:"(w23) -> ()
          n54 = local write "Mail Test Fail"(w21) -> ()
          n55 = local write "Fail Loops"(w29) -> ()
          n56 = local write "Temp Delay Lps"(w32) -> ()
          n57 = local write "C drive data root dir"(w41) -> ()
          n58 = local write "Temp Value"(w31) -> ()
          n59 = local write "Network Directory"(w43) -> ()
          n60 = local write "SAMPLES"(w37) -> ()
          n61 = local write "RATE (Hz)"(w36) -> ()
          n62 = local write "SET LAB04-2"(w46) -> ()
          n63 = local write "SET LAB05-1"(w45) -> ()
          n64 = local write "SET LAB04-1"(w47) -> ()
          n65 = local write "SET LAB05-2"(w44) -> ()
          n66 = local write "SET LAB02-1"(w51) -> ()
          n67 = local write "SET LAB02-2"(w50) -> ()
          n68 = local write "SET LAB03-1"(w49) -> ()
          n69 = local write "SET LAB03-2"(w48) -> ()
          n70 = local write "SET LAB01-1"(w53) -> ()
          n71 = local write "SET LAB01-2"(w52) -> ()
          n72 = local write "Select COM port"(w20) -> ()
          n73 = global write "Global 1.vi" "COM port"(w20) -> ()
        }
        frame #5 {
          # "Get total resets value from file"
          n74 = String To Path(string="c:\\crabtree\\Set Up\\") -> (path=w86:path)
          n75 = Build Path(base path=w86, name or relative path="USB resets.bin") -> (appended path=w79:path)
          n76 = Create Folder(path (use dialog)=w86) -> (error out=w78:errorcluster)  [unwired: 2 in, 2 out]
          n77 = call <vilib>:"Clear Errors.vi"("error in (no error)"=w78) -> ()  [unwired: 5 in, 2 out]
          n78 = Open/Create/Replace File(file path (use dialog)=w79, operation (0:open)=T18."open or create") -> (refnum out=w84:refnum<file>, error out=w83:errorcluster)  [unwired: 4 in, 1 out]
          n79 = local read "Total USB resets"() -> (w77:dbl)
          n80 = Read from Binary File(5:w77, 8:w83, 11:w84) -> (0:w81:errorcluster, 2:w76:dbl, 3:w82:refnum<file>)  [unwired: 3 in, 1 out]
          n81 = local write "Total USB resets"(w76) -> ()
          n82 = Close File(refnum=w82, error in=w81) -> (error out=w80:errorcluster)  [unwired: 1 out]
          n83 = local write "data file error"(w80) -> ()
        }
        frame #6 {
          # "Get last saved jig cycles value from file"
          n84 = String To Path(string="c:\\crabtree\\Jig Cycles\\") -> (path=w98:path)
          n85 = Build Path(base path=w98, name or relative path="jigcycles.bin") -> (appended path=w96:path)
          n86 = Create Folder(path (use dialog)=w98) -> (error out=w100:errorcluster)  [unwired: 2 in, 2 out]
          n87 = call <vilib>:"Clear Errors.vi"("error in (no error)"=w100) -> ()  [unwired: 5 in, 2 out]
          n88 = Open/Create/Replace File(file path (use dialog)=w96) -> (refnum out=w94:refnum<file>, error out=w95:errorcluster)  [unwired: 5 in, 1 out]
          n89 = Read from Binary File(5:T9 {"LAB01-1"=0.0, "LAB01-2"=0.0, "LAB02-1"=0.0, "LAB02-2"=0.0, "LAB03-1"=0.0, "LAB03-2"=0.0, "LAB04-1"=0.0, "LAB04-2"=0.0, "LAB05-1"=0.0, "LAB05-2"=0.0} ("JIG RELAY CYCLES"), 8:w95, 11:w94) -> (0:w92:errorcluster, 2:w89:T9, 3:w93:refnum<file>)  [unwired: 3 in, 1 out]
          n90 = local write "JIG RELAY CYCLES"(w89) -> ()
          n91 = Close File(refnum=w93, error in=w92) -> (error out=w91:errorcluster)  [unwired: 1 out]
          n92 = local write "data file error"(w91) -> ()
        }
        frame #7 {
          # "Get mail settings"
          n93 = local read "Auto Mail Send"() -> (w104:bool)
          n94 = local read "MAIL SETTINGS"() -> (w108:T8)
          n95 = String To Path(string="c:\\crabtree\\Set Up\\") -> (path=w116:path)
          n96 = Build Path(base path=w116, name or relative path="mail.bin") -> (appended path=w114:path)
          n97 = Create Folder(path (use dialog)=w116) -> (error out=w118:errorcluster)  [unwired: 2 in, 2 out]
          n98 = Bundle("MAIL SETTINGS"=w108, "Auto Mail Send"=w104, "") -> (w107:T25)  [unwired: 1 in]
          n99 = call <vilib>:"Clear Errors.vi"("error in (no error)"=w118) -> ()  [unwired: 5 in, 2 out]
          n100 = Open/Create/Replace File(file path (use dialog)=w114) -> (refnum out=w112:refnum<file>, error out=w113:errorcluster)  [unwired: 5 in, 1 out]
          n101 = Read from Binary File(5:w107, 8:w113, 11:w112) -> (0:w110:errorcluster, 2:w106:T25, 3:w111:refnum<file>)  [unwired: 3 in, 1 out]
          n102 = Unbundle(w106) -> ("MAIL SETTINGS"=w105:T8, "Auto Mail Send"=w103:bool, w102:string)
          n103 = local write "Auto Mail Send"(w103) -> ()
          n104 = local write "TO (string):"(w102) -> ()
          n105 = local write "MAIL SETTINGS"(w105) -> ()
          n106 = Close File(refnum=w111, error in=w110) -> (error out=w109:errorcluster)  [unwired: 1 out]
          n107 = local write "data file error"(w109) -> ()
        }
        frame #8 {
          # "Set display status if blank"
          n108 = local read "DISP LAB03-2"() -> (w148:T4)
          n109 = local read "DISP LAB03-1"() -> (w155:T4)
          n110 = local read "DISP LAB02-2"() -> (w162:T4)
          n111 = local read "DISP LAB01-2"() -> (w175:T4)
          n112 = local read "DISP LAB01-1"() -> (w184:T4)
          n113 = local read "DISP LAB02-1"() -> (w169:T4)
          n114 = Unbundle(w148) -> ("STATUS"=w150:string)  [unwired: 2 out]
          n115 = Unbundle(w155) -> ("STATUS"=w157:string)  [unwired: 2 out]
          n116 = Unbundle(w162) -> ("STATUS"=w164:string)  [unwired: 2 out]
          n117 = Unbundle(w169) -> ("STATUS"=w171:string)  [unwired: 2 out]
          n118 = Unbundle(w175) -> ("STATUS"=w178:string)  [unwired: 2 out]
          n119 = Unbundle(w184) -> ("STATUS"=w185:string)  [unwired: 2 out]
          n120 = Equal?(x="", y=w150) -> (x = y?=w152:bool)
          n121 = Equal?(x="", y=w157) -> (x = y?=w159:bool)
          n122 = Equal?(x="", y=w164) -> (x = y?=w166:bool)
          n123 = Equal?(x="", y=w171) -> (x = y?=w173:bool)
          n124 = Equal?(x="", y=w178) -> (x = y?=w180:bool)
          n125 = Equal?(x="", y=w185) -> (x = y?=w187:bool)
          n126 = Select(t="STOP", s=w152, f=w150) -> (s? t:f=w149:string)
          n127 = Select(t="STOP", s=w159, f=w157) -> (s? t:f=w156:string)
          n128 = Select(t="STOP", s=w166, f=w164) -> (s? t:f=w163:string)
          n129 = Select(t="STOP", s=w173, f=w171) -> (s? t:f=w170:string)
          n130 = Select(t="STOP", s=w180, f=w178) -> (s? t:f=w177:string)
          n131 = Select(t="STOP", s=w187, f=w185) -> (s? t:f=w183:string)
          n132 = Bundle(cluster=w148, "STATUS"=w149) -> (w147:T4)  [unwired: 2 in]
          n133 = Bundle(cluster=w155, "STATUS"=w156) -> (w154:T4)  [unwired: 2 in]
          n134 = Bundle(cluster=w162, "STATUS"=w163) -> (w161:T4)  [unwired: 2 in]
          n135 = Bundle(cluster=w169, "STATUS"=w170) -> (w168:T4)  [unwired: 2 in]
          n136 = Bundle(cluster=w175, "STATUS"=w177) -> (w176:T4)  [unwired: 2 in]
          n137 = Bundle(cluster=w184, "STATUS"=w183) -> (w182:T4)  [unwired: 2 in]
          n138 = local write "DISP LAB01-2"(w176) -> ()
          n139 = local write "DISP LAB01-1"(w182) -> ()
          n140 = local write "DISP LAB02-1"(w168) -> ()
          n141 = local write "DISP LAB03-1"(w154) -> ()
          n142 = local write "DISP LAB02-2"(w161) -> ()
          n143 = local write "DISP LAB03-2"(w147) -> ()
          n144 = local read "DISP LAB05-2"() -> (w120:T4)
          n145 = local read "DISP LAB05-1"() -> (w127:T4)
          n146 = local read "DISP LAB04-2"() -> (w129:T4)
          n147 = local read "DISP LAB04-1"() -> (w131:T4)
          n148 = Unbundle(w120) -> ("STATUS"=w122:string)  [unwired: 2 out]
          n149 = Unbundle(w127) -> ("STATUS"=w133:string)  [unwired: 2 out]
          n150 = Unbundle(w129) -> ("STATUS"=w138:string)  [unwired: 2 out]
          n151 = Unbundle(w131) -> ("STATUS"=w143:string)  [unwired: 2 out]
          n152 = Equal?(x="", y=w122) -> (x = y?=w124:bool)
          n153 = Equal?(x="", y=w133) -> (x = y?=w135:bool)
          n154 = Equal?(x="", y=w138) -> (x = y?=w140:bool)
          n155 = Equal?(x="", y=w143) -> (x = y?=w145:bool)
          n156 = Select(t="STOP", s=w124, f=w122) -> (s? t:f=w121:string)
          n157 = Select(t="STOP", s=w135, f=w133) -> (s? t:f=w132:string)
          n158 = Select(t="STOP", s=w140, f=w138) -> (s? t:f=w137:string)
          n159 = Select(t="STOP", s=w145, f=w143) -> (s? t:f=w142:string)
          n160 = Bundle(cluster=w120, "STATUS"=w121) -> (w119:T4)  [unwired: 2 in]
          n161 = Bundle(cluster=w127, "STATUS"=w132) -> (w126:T4)  [unwired: 2 in]
          n162 = Bundle(cluster=w129, "STATUS"=w137) -> (w128:T4)  [unwired: 2 in]
          n163 = Bundle(cluster=w131, "STATUS"=w142) -> (w130:T4)  [unwired: 2 in]
          n164 = local write "DISP LAB05-2"(w119) -> ()
          n165 = local write "DISP LAB05-1"(w126) -> ()
          n166 = local write "DISP LAB04-1"(w130) -> ()
          n167 = local write "DISP LAB04-2"(w128) -> ()
        }
        frame #9 {
          w192 = 0
          w189 = FALSE
          # "initialise analog error control"
          n168 = local write "Resets Done"(0) -> ()
          n169 = local write "Auto Reset"(TRUE) -> ()
          n170 = local write "Er USB#0"(w192) -> ()
          n171 = local write "Er USB#1"(w192) -> ()
          n172 = local write "Er USB#2"(w192) -> ()
          n173 = local write "Analog error"(w189) -> ()
          n174 = local write "Reset Measuring"(w189) -> ()
          n175 = local write "Error USB #0"(w189) -> ()
          n176 = local write "Reset Error"(w189) -> ()
          n177 = local write "Error USB #1"(w189) -> ()
          n178 = local write "Error USB #2"(w189) -> ()
          n179 = local write "stop"(w189) -> ()
          n180 = local write "stop all"(w189) -> ()
        }
        frame #10 {
          # "get initial temperature values"
          n181 = stacked-sequence {
            frame #0 {
              w201 = T13 {"T1 Live"=20.0, "T1 Neut"=20.0, "T2 Live"=20.0, "T2 Neut"=20.0, "ID"=6.0, "ER"=10.0} ("LAB01 TEMP")
              n182 = local read "Select COM port"() -> (w196:refnum<visa-resource-name>)
              n183 = local write "LAB deg C"(w201) -> ()
              n184 = global write "Global display 4.vi" "LAB deg C"(w201) -> ()
              n185 = local write "OFF amps"(1.5) -> ()
              n186 = local write "ON amps"(20.0) -> ()
              n187 = local write "VOLTS"(250.0) -> ()
              n188 = local write "PF"(0.5) -> ()
              n189 = call "sub vi-open serial port v1.vi"("Select COM port"=w196) -> ("Error"=→"Com Port Status":bool, "LOOPS"=→"Com setup loops":i32, "VISA Com out"=→"VISA Com out":refnum<visa-resource-name>)  [unwired: 12 in]
            }
            frame #1 {
              n190 = for {
